vi "createEvnts.vi"(8 "error in (no error)":errorcluster, 11 "Electrometer in":refnum<class "Electrometer.lvclass">) -> (0 "error out":errorcluster, 3 "Electrometer out":refnum<class "Electrometer.lvclass">)   [LabVIEW 2016, in "Electrometer.lvclass"]
uses:
  Electrometer.lvclass
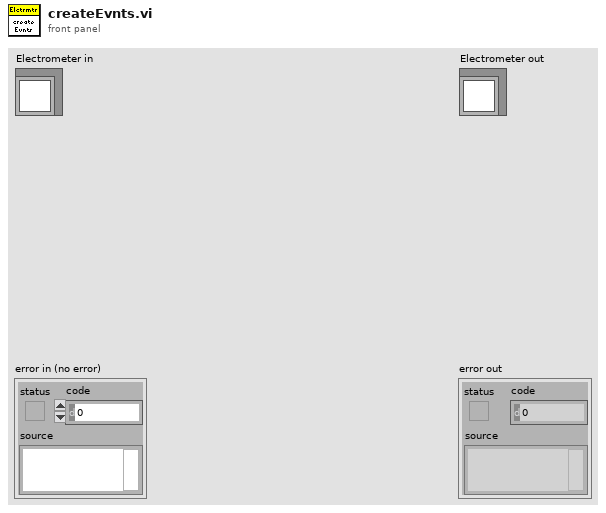
[diagram p1: front panel]
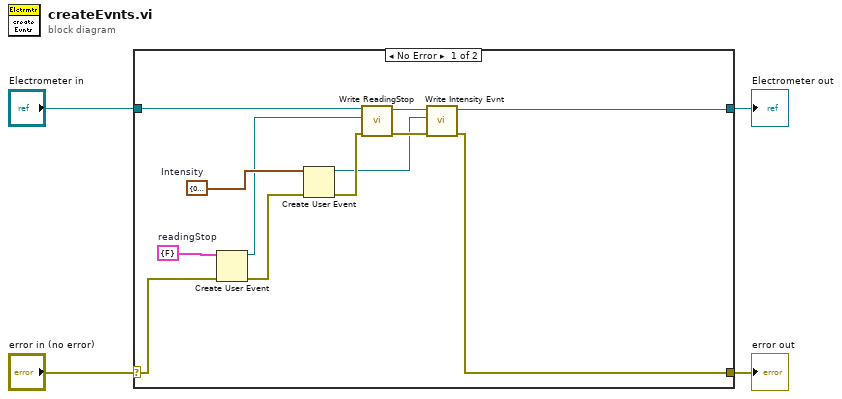
[diagram p0: block diagram]
diagram:
  n1 = case shown="No Error" "error in (no error)" {
    selector: "error in (no error)" -> [w14 w18]
    tunnel: [w6 w18] -> w3
    tunnel: [w5 w17] -> w1
    tunnel: "Electrometer in" -> [w13 w17]
    frame No Error {
      w15 = cluster{"stop":bool} {"stop"=FALSE}  # readingStop
      w16 = cluster{"Intensity":dbl, "id":dbl} {"Intensity"=0.0, "id"=0.0}  # Intensity
      n2 = Create User Event(user event datatype=w15, error in=w14) -> (user event=w12:refnum<user-event>, error out=w11:errorcluster)
      n3 = Create User Event(user event datatype=w16, error in=w11) -> (user event=w7:refnum<user-event>, error out=w8:errorcluster)
      n4 = call-dynamic "Write ReadingStop.vi"("error in (no error)"=w8, "ReadingStop"=w12, "Electrometer in"=w13) -> ("error out"=w9:errorcluster, "Electrometer out"=w10:refnum<class "Electrometer.lvclass">)  [unwired: 7 in]
      n5 = call-dynamic "Write Intensity Evnt.vi"("error in (no error)"=w9, "IntensityEvnt"=w7, "Electrometer in"=w10) -> ("error out"=w6:errorcluster, "Electrometer out"=w5:refnum<class "Electrometer.lvclass">)  [unwired: 7 in]
    }
    frame Error {
    }
  }
  "error out" <- w3
  "Electrometer out" <- w1
